vi "Schritt2.vi"() -> ()   [LabVIEW 2009]
uses:
  Vibe/Delta_t.vi
panel:
  out "Druck [bar]":ext[](array[numeric])
  in  "5. Befüllschritt":u16(ring) items=["H2", "CH4", "C2H2", "O2", "N2"]
  in  "4. Befüllschritt":u16(ring) items=["H2", "CH4", "C2H2", "O2", "N2"]
  in  "3. Befüllschritt":u16(ring) items=["H2", "CH4", "C2H2", "O2", "N2"]
  in  "2. Befüllschritt":u16(ring) items=["H2", "CH4", "C2H2", "O2", "N2"]
  in  "1. Befüllschritt":u16(ring) items=["H2", "CH4", "C2H2", "O2", "N2"]
  in  "Wandtemperatur [K]":dbl
  in  "Brenndauer":dbl
  out "T(t)":dbl[](graph)
  in  "T0":dbl format="%.2f"
  in  "dt":dbl
  in  "Startzeit":dbl
  in  "Stoppzeit":dbl
  in  "Molmasse C":dbl min=12.0 max=12.0
  in  "Molmasse C2H2":dbl min=26.0 max=26.0
  in  "Molmasse CH4":dbl min=16.0 max=16.0
  in  "Molmasse CO2":dbl min=44.0 max=44.0
  in  "Molmasse N2":dbl min=28.0 max=28.0
  in  "Molmasse O2":dbl min=32.0 max=32.0
  in  "Molmasse H2O":dbl min=18.0 max=18.0
  in  "Molmasse H2":dbl min=2.0 max=2.0
  in  "Verdichtungsverhältnis":dbl
  in  "Anzahl Zylinder [Stück]":dbl min=0.0
  in  "Hubraum [m^3]":dbl
  in  "Kammervolumen [m^3]":dbl
  in  "Lambda Luft":dbl
  in  "Brennstoffmasse [g/Arbeitsspiel]":dbl
  in  "o":dbl min=0.0 max=1.0 step=0.01
  in  "h":dbl min=0.0 max=1.0 step=0.01
  in  "c":dbl min=0.0 max=1.0 step=0.01
  in  "AGR- Rate":dbl(knob) min=0.01 max=0.9 step=0.01
  # "Verbrennungseinstellungen"
  # "Kraftstoffdaten"
  # "Notwendig!"
  # "Molmassen [g/mol]"
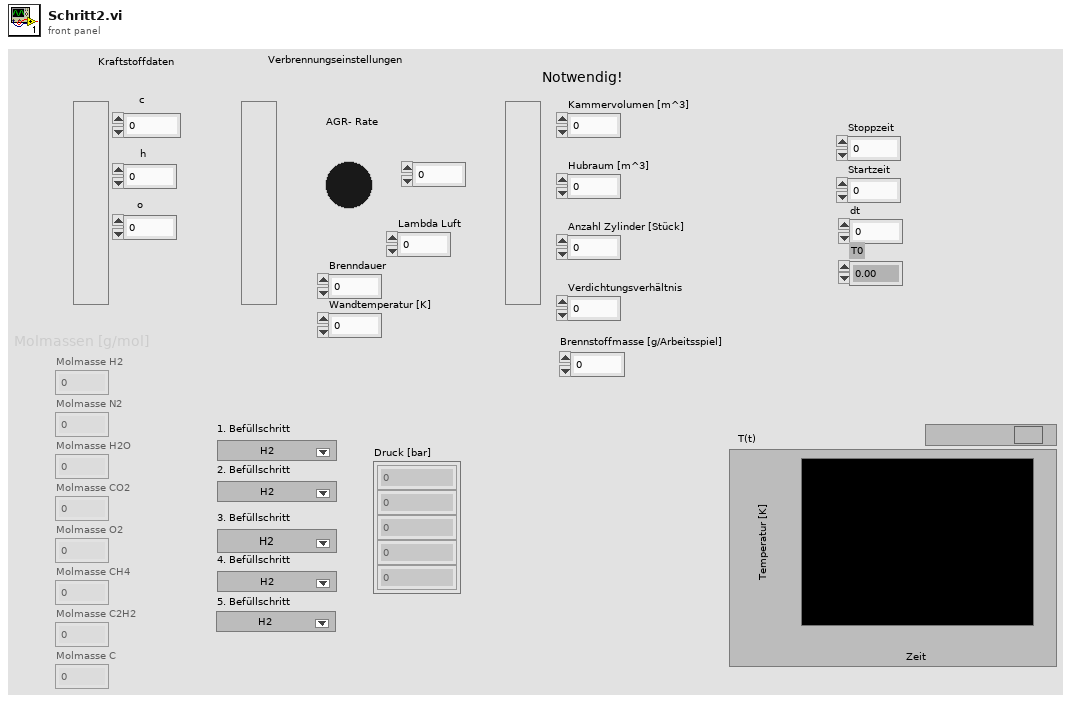
[diagram p1: front panel]
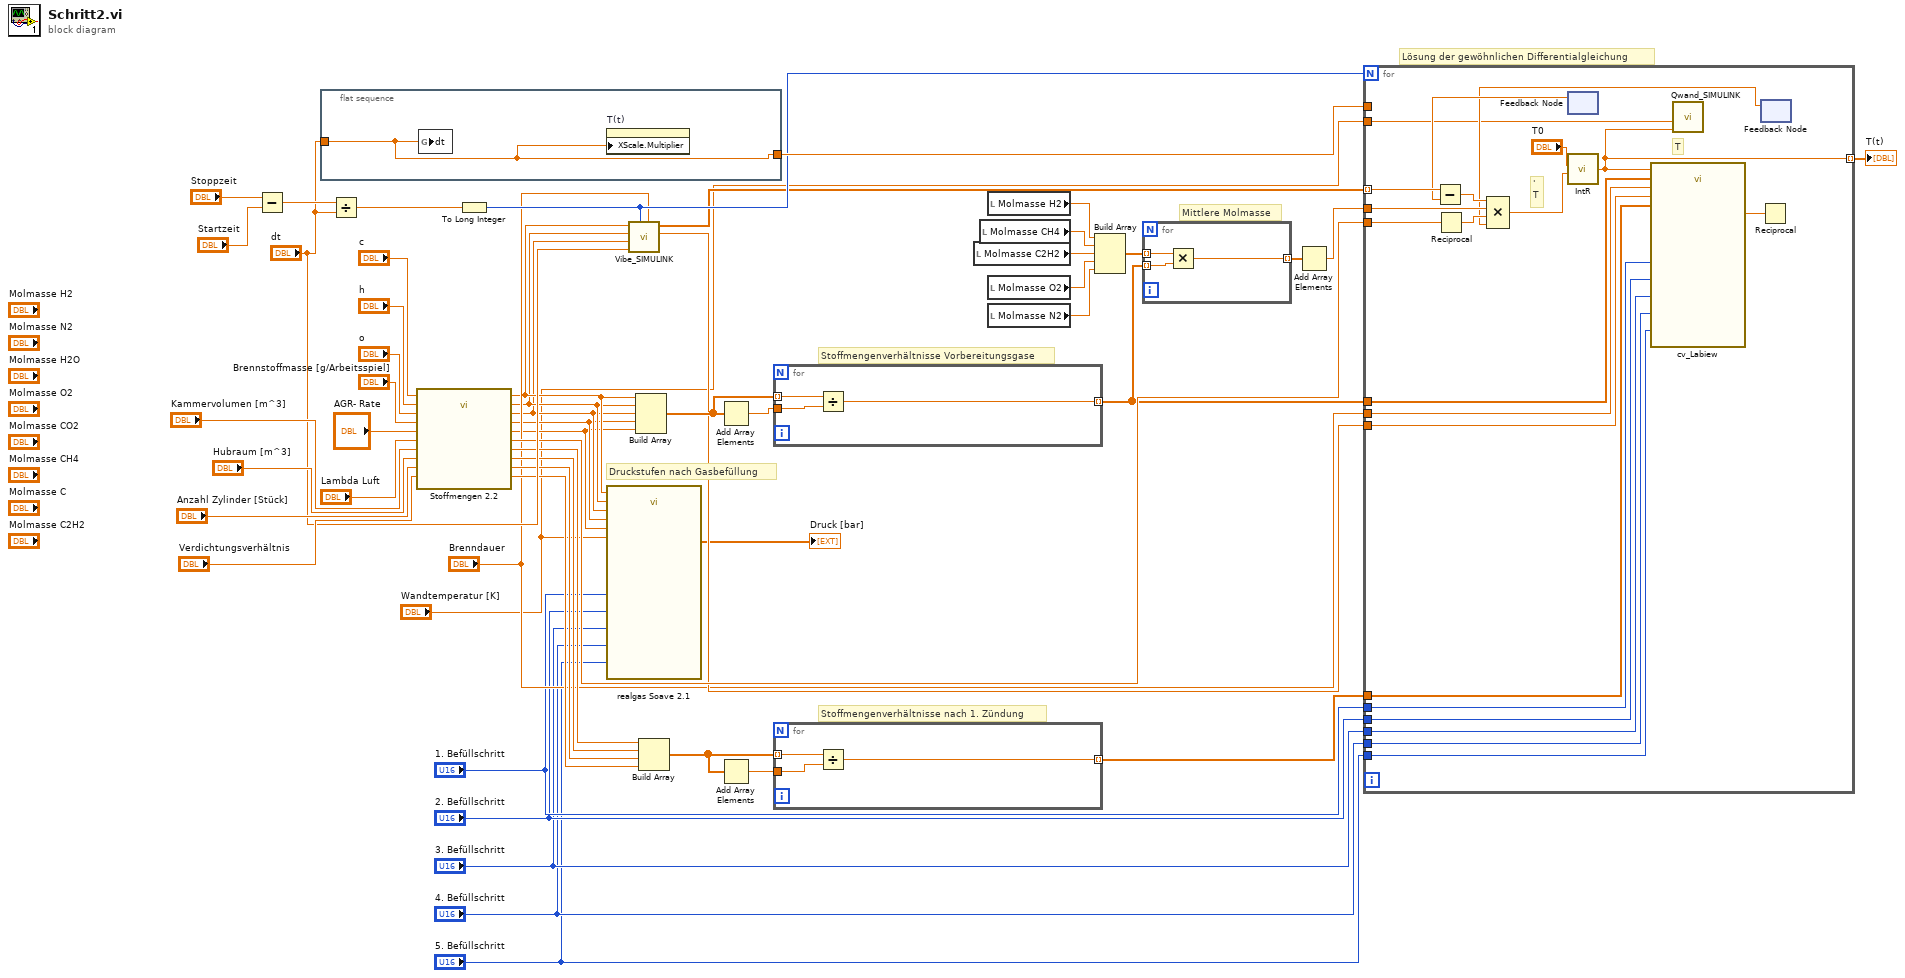
[diagram p0: block diagram]
diagram:
  # "Druckstufen nach Gasbefüllung"
  # "Stoffmengenverhältnisse nach 1. Zündung"
  # "Lösung der gewöhnlichen Differentialgleichung"
  # "Mittlere Molmasse"
  # "Stoffmengenverhältnisse Vorbereitungsgase"
  n1 = Subtract(x="Stoppzeit", y="Startzeit") -> (x-y=w31:dbl)
  n2 = flat-sequence {
    tunnel: "dt" -> [w53]
    tunnel: [w53] -> w30
    frame #0 {
      n3 = global write "Delta_t.vi" "dt"(w53) -> ()
      n4 = property on="T(t)" class="SVGraph (strikt)"("XScale.Multiplier"=w53) -> ()  [unwired: 2 in, 2 out]
    }
  }
  n5 = Divide(x=w31, y="dt") -> (x/y=w29:dbl)
  n6 = call "Stoffmengen 2.2.vi"("c"="c", "h"="h", "o"="o", "Brennstoffmasse [g/Arbeitsspiel]"="Brennstoffmasse [g/Arbeitsspiel]", "AGR- Rate"="AGR- Rate", "Lambda Luft"="Lambda Luft", "Kammervolumen [m^3]"="Kammervolumen [m^3]", "Hubraum [m^3]"="Hubraum [m^3]", "Verdichtungsverhältnis"="Verdichtungsverhältnis", "Anzahl Zylinder [Stück]"="Anzahl Zylinder [Stück]") -> ("nO2,Kammer"=w17:dbl, "nH2O,Kammer"=w18:dbl, "nN2,Kammer"=w16:dbl, "nCO2,Kammer"=w19:dbl, "H2 [mol]"=w12:dbl, "CH4 [mol]"=w11:dbl, "C2H2 [mol]"=w10:dbl, "O2 [mol]"=w9:dbl, "N2 [mol]"=w8:dbl, "Masse in Kammer [g]"=w25:dbl)  [unwired: 7 in, 1 out]
  n7 = To Long Integer(number=w29) -> (32bit integer=w27:i32)
  n8 = call "realgas Soave 2.1.vi"("Stoffmenge H2 [mol]"=w12, "Stoffmenge CH4 [mol]"=w11, "Stoffmenge C2H2 [mol]"=w10, "Stoffmenge O2 [mol]"=w9, "Stoffmenge N2 [mol]"=w8, "T [K]"="Wandtemperatur [K]", "1. Befüllschritt"="1. Befüllschritt", "4. Befüllschritt"="4. Befüllschritt", "2. Befüllschritt"="2. Befüllschritt", "5. Befüllschritt"="5. Befüllschritt", "3. Befüllschritt"="3. Befüllschritt") -> ("Druck [bar]"=→"Druck [bar]":ext[])  [unwired: 16 in]
  n9 = call "Vibe_SIMULINK.vi"("Brenndauer"="Brenndauer", "Iterationsschritte"=w27, "dt"="dt", "C2H2 [mol]"=w10, "CH4 [mol]"=w11, "H2 [mol]"=w12) -> ("Aktuelle Zeit"=w15:dbl, "Array"=w22:dbl[])  [unwired: 4 in]
  n10 = Build Array(w12, w11, w10, w9, w8) -> (w42:dbl[])
  n11 = Build Array(w19, w18, w17, w16) -> (w20:dbl[])
  n12 = Add Array Elements(numeric array=w42) -> (sum=w41:dbl)
  n13 = Add Array Elements(numeric array=w20) -> (sum=w21:dbl)
  n14 = for {
    tunnel: w42 -> [w56] mode=indexing
    tunnel: w41 -> [w55]
    tunnel: [w54] -> w24 mode=indexing
    n15 = Divide(x=w56, y=w55) -> (x/y=w54:dbl)
  }
  n16 = for {
    tunnel: w20 -> [w59] mode=indexing
    tunnel: w21 -> [w58]
    tunnel: [w57] -> w13 mode=indexing
    n17 = Divide(x=w59, y=w58) -> (x/y=w57:dbl)
  }
  n18 = local read "Molmasse C2H2"() -> (w34:dbl)
  n19 = local read "Molmasse CH4"() -> (w40:dbl)
  n20 = local read "Molmasse H2"() -> (w39:dbl)
  n21 = local read "Molmasse O2"() -> (w38:dbl)
  n22 = local read "Molmasse N2"() -> (w37:dbl)
  n23 = Build Array(w39, w40, w34, w38, w37) -> (w36:dbl[])
  n24 = for {
    tunnel: w24 -> [w61] mode=indexing
    tunnel: w36 -> [w62] mode=indexing
    tunnel: [w60] -> w35 mode=indexing
    n25 = Multiply(x=w62, y=w61) -> (x*y=w60:dbl)
  }
  n26 = Add Array Elements(numeric array=w35) -> (sum=w26:dbl)
  n27 = for {
    N: w27 -> [_]
    tunnel: w30 -> [_]
    tunnel: w22 -> [w85] mode=indexing
    tunnel: w26 -> [w77]
    tunnel: w25 -> [w76]
    tunnel: w24 -> [w79]
    tunnel: [w72] -> w23 mode=indexing
    tunnel: w15 -> [w70]
    tunnel: "Brenndauer" -> [w71]
    tunnel: w13 -> [w69]
    tunnel: "Wandtemperatur [K]" -> [w68]
    tunnel: "1. Befüllschritt" -> [w67]
    tunnel: "2. Befüllschritt" -> [w66]
    tunnel: "3. Befüllschritt" -> [w65]
    tunnel: "4. Befüllschritt" -> [w64]
    tunnel: "5. Befüllschritt" -> [w63]
    # "T"
    # "'\nT"
    n28 = Reciprocal(x=w76) -> (1/x=w75:dbl)
    n29 = feedback #1() -> (w78:dbl)  [unwired: 1 in]
    n30 = Subtract(x=w85, y=w78) -> (x-y=w84:dbl)
    n31 = feedback #2() -> (w74:dbl)  [unwired: 1 in]
    n32 = Compound Arithmetic op=MULTIPLY(w84, w77, w75, w74) -> (w83:dbl)
    n33 = call "IntR.vi"("xpunkt(t)"=w83, "x0"="T0") -> ("x(t)"=w72:dbl)  [unwired: 2 in]
    n34 = call "cv_Labiew.vi"("T [K]"=w72, "1. Befüllschritt"=w67, "2. Befüllschritt"=w66, "3. Befüllschritt"=w65, "Stoffmengenverhältnisse Vorbereitungsgase"=w79, "Brenndauer"=w71, "Aktuelle Zeit"=w70, "Stoffmengenverhältnisse Gase nach 1. Verbrennung"=w69, "4. Befüllschritt"=w64, "5. Befüllschritt"=w63) -> ("cv"=w81:dbl)  [unwired: 5 in]
    n35 = call "Qwand_SIMULINK.vi"("Temperatur [K]"=w72, "Wandtemperatur [K]"=w68) -> ("Qw"=w73:dbl)  [unwired: 9 in]
    n36 = Reciprocal(x=w81) -> (1/x=w80:dbl)
  }
  "T(t)" <- w23
